vi "Teleop.vi"(10 "Match Info":T1={"Autonomous Elapsed Seconds"=0.0, "TeleOp Elapsed Seconds"=0.0, "Disabled Elapsed Seconds"=0.0, "Visited Autonomous"=FALSE, "Visited TeleOp"=FALSE, "Visited Disabled"=FALSE, "Autonomous Settings"={"Autonomous Style"=enum."Independent", "VI Refnum"=refnum}}, 11 "Call Context":T2) -> ()   [LabVIEW 2017]
doc: "This VI is called for each TeleOp packet received from the DS where the robot is not disabled. It is often used to read from the joysticks and update I/O or to update setpoints for timed control loops. It should complete and return within 20 milliseconds or it may miss DS packets."
uses:
  <vilib>/Rock Robotics/WPI/DriverStation/WPI_DriverStationDerivedRobotMode.ctl
  <vilib>/Rock Robotics/WPI/DriverStation/WPI_DriverStationMatch Info.ctl
  <vilib>/Rock Robotics/WPI/Solenoid/WPI_SolenoidValue.ctl
  <vilib>/Rock Robotics/WPI/ThirdParty/Phoenix-LabVIEW/Motor Controller/Controls/CTRE_Phoenix_MotorControl_ControlMode.ctl
  <vilib>/Rock Robotics/WPI/Utilities/WPI_GetSetVariantRefNum.vi
  <vilib>/Rock Robotics/WPI/Solenoid/WPI_SolenoidSetEnum.vi
  <vilib>/Rock Robotics/Network Tables/NT Write Boolean Array.vi
  <vilib>/Rock Robotics/Network Tables/NT Write Numeric Array.vi
  <vilib>/Rock Robotics/Network Tables/NT Read Boolean.vi
  <vilib>/Rock Robotics/Network Tables/NT Read Number.vi
  Robot Global Data.vi
  <vilib>/addons/control/pid/NI_PID_pid.lvlib
  <vilib>/addons/control/pid/pid.llb/PID (DBL).vi
panel:
  out "AbsArm":dbl
  out "Sample Slider 0":dbl(slide) scale=0.0..5.0
  out "Sample Boolean 1":bool
  out "Sample Boolean 0":bool
  # "TUSKS"
  # "Axis 1"
  # "DRIVE"
  # "Axis 1"
  # "PULSE"
  # "Button 3"
  # "Button 3"
  # "Axis 0"
  # "Axis 0"
  # "Button 2"
  # "Button 1"
  # "Button 2"
  # "Button 1"
  # "Button 0"
  # "Button 0"
  # "CONTROLLER  LAYOUT"
  # "CONTROLLER  LAYOUT"
  # "Joystick 1"
  # "Joystick 0"
  # "Joystick 1"
  # "https://www.xbox.com/en-us/xbox-one/accessories"
  # "Axis 4"
  # "Axis 4"
  # "DRIVE TURN"
  # "Left"
  # "Left"
  # "Axis 5"
  # "Axis 5"
  # "CLAW IN"
  # "Button 4"
  # "ELBOW DOWN"
  # "Button 4"
  # "Axis 2"
  # "ARM DOWN"
  # "Axis 2"
  # "BELT IN"
  # "Right"
  # "Button 5"
  # "ELBOW UP"
  # "Button 5"
  # "CLAW OUT"
  # "Axis 3"
  # "ARM UP"
  # "Axis 3"
  # "BELT OUT"
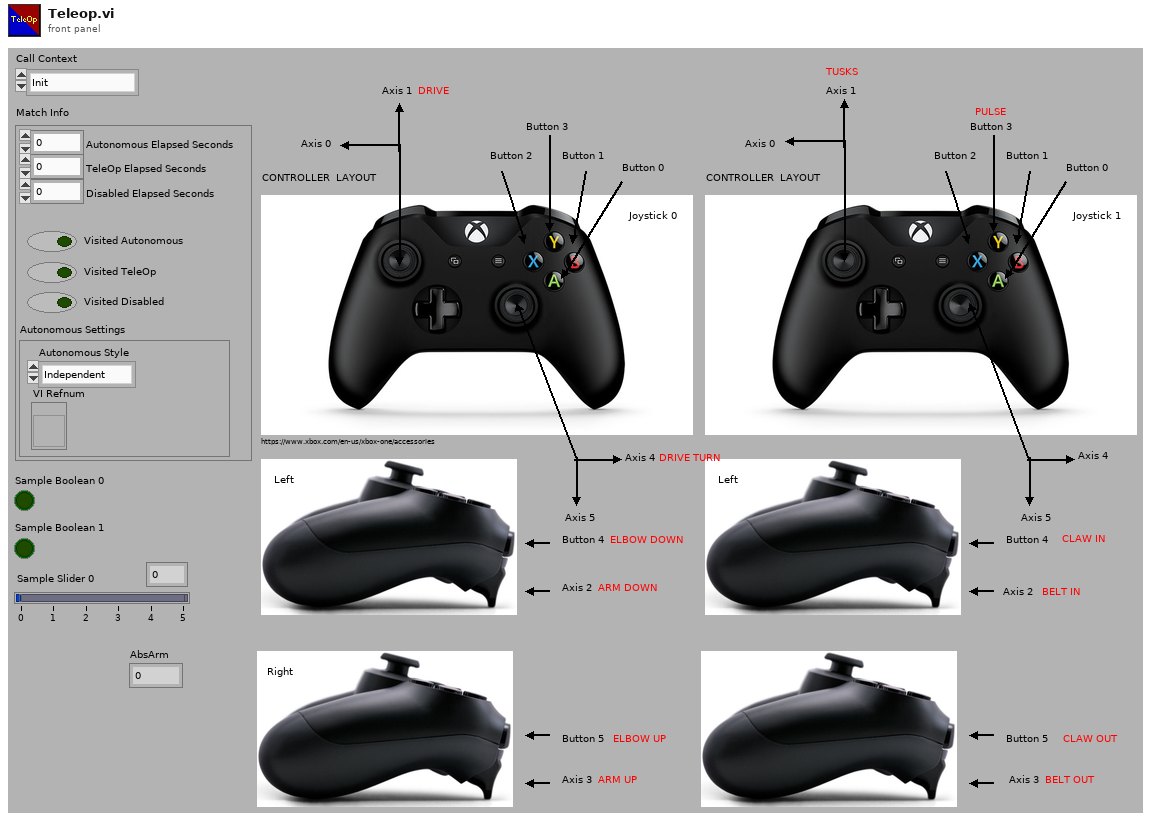
[diagram p1: front panel]
types:
  T1 = typedef "WPI_DriverStationMatch Info.ctl" = cluster{"Autonomous Elapsed Seconds":dbl, "TeleOp Elapsed Seconds":dbl, "Disabled Elapsed Seconds":dbl, "Visited Autonomous":bool, "Visited TeleOp":bool, "Visited Disabled":bool, "Autonomous Settings":cluster{"Autonomous Style":enum16{"Iterative", "Independent"}, "VI Refnum":refnum<vi>}}
  T2 = typedef "WPI_DriverStationDerivedRobotMode.ctl" = enum16{"Init", "Execute", "Stop"}
  T3 = typedef "WPI_JoystickDevRef.ctl" = cluster{"Device":T4}
  T4 = typedef "WPI_JoystickDeviceEnum.ctl" = enum16{"USB 0", "USB 1", "USB 2", "USB 3", "USB 4", "USB 5"}
  T5 = cluster{"Axes[0]":dbl, "Axes[1]":dbl, "Axes[2]":dbl, "Axes[3]":dbl, "Axes[4]":dbl, "Axes[5]":dbl, "Axes[6]":dbl, "Axes[7]":dbl, "Axes[8]":dbl}
  T6 = cluster{"Buttons[0]":bool, "Buttons[1]":bool, "Buttons[2]":bool, "Buttons[3]":bool, "Buttons[4]":bool, "Buttons[5]":bool, "Buttons[6]":bool, "Buttons[7]":bool, "Buttons[8]":bool}
  T7 = typedef "CTRE_Phoenix_MotorControl_ControlMode.ctl" = u16
  T8 = typedef "WPI_MotorControlDeviceRef.ctl" = cluster{"DeviceStatus":errorcluster, "Type":T9, "PWM":cluster{"PWM Channel":T10, "DeadBand":T11}, "CAN":cluster{"Device Number":u8, "SetOutput VI Ref":variant, "GetOutput VI Ref":variant, "Enable VI Ref":variant, "Disable VI Ref":variant, "Data":variant}, "Invert":bool, "DIO PWM":cluster{"PWM \"Enable\" Channel":T10, "DIOChannel":T12, "PWM Rate":dbl}}
  T9 = typedef "WPI_MotorControlType.ctl" = enum16{"PWM", "CAN", "DIO PWM"}
  T10 = typedef "FPGA_DIOPWMChannel.ctl" = enum8{"PWM 0", "PWM 1", "PWM 2", "PWM 3", "PWM 4", "PWM 5", "PWM 6", "PWM 7", "PWM 8", "PWM 9", "PWM MXP 0", "PWM MXP 1", "PWM MXP 2", "PWM MXP 3", "PWM MXP 4", "PWM MXP 5", "PWM MXP 6", "PWM MXP 7", "PWM MXP 8", "PWM MXP 9", "Invalid"}
  T11 = typedef "WPI_PWMDeadband.ctl" = cluster{"Name":string, "maxPositivePwm":i32, "minPositivePwm":i32, "centerPwm":i32, "maxNegativePwm":i32, "minNegativePwm":i32, "angularRange":u16}
  T12 = typedef "FPGA_DIOChannel.ctl" = enum8{"DIO 0", "DIO 1", "DIO 2", "DIO 3", "DIO 4", "DIO 5", "DIO 6", "DIO 7", "DIO 8", "DIO 9", "DIO MXP 0", "DIO MXP 1", "DIO MXP 2", "DIO MXP 3", "DIO MXP 4", "DIO MXP 5", "DIO MXP 6", "DIO MXP 7", "DIO MXP 8", "DIO MXP 9", "DIO MXP 10", "DIO MXP 11", "DIO MXP 12", "DIO MXP 13", "DIO MXP 14", "DIO MXP 15", "SPI Port CS1", "SPI Port CS2", "SPI Port CS3", "SPI Port MISO", "SPI Port MOSI", "Invalid"}
  T13 = enum16{"Arm Down", "Arm Switch", "Arm(Low Scale)", "Arm(Normal Scale)", "Arm(High Scale)", "Hang"}
  T14 = cluster{"proportional gain (Kc)":dbl, "integral time (Ti, min)":dbl, "derivative time (Td, min)":dbl}
  T15 = enum16{"Arm Down", "Arm Switch", "Arm(Low Scale)", "Arm(Normal Scale)", "Arm(High Scale)"}
  T16 = typedef "WPI_SolenoidValue.ctl" = enum16{"Off", "On", "Forward", "Reverse"}
  T17 = typedef "WPI_SolenoidDevRef.ctl" = cluster{"DevStatus":errorcluster, "Pneumatics Control Module":u8, "Forward Solenoid Channel":T18, "Reverse Solenoid Channel":T18}
  T18 = typedef "WPI_SolenoidChannel.ctl" = enum8{"Solenoid 0", "Solenoid 1", "Solenoid 2", "Solenoid 3", "Solenoid 4", "Solenoid 5", "Solenoid 6", "Solenoid 7", "Invalid"}
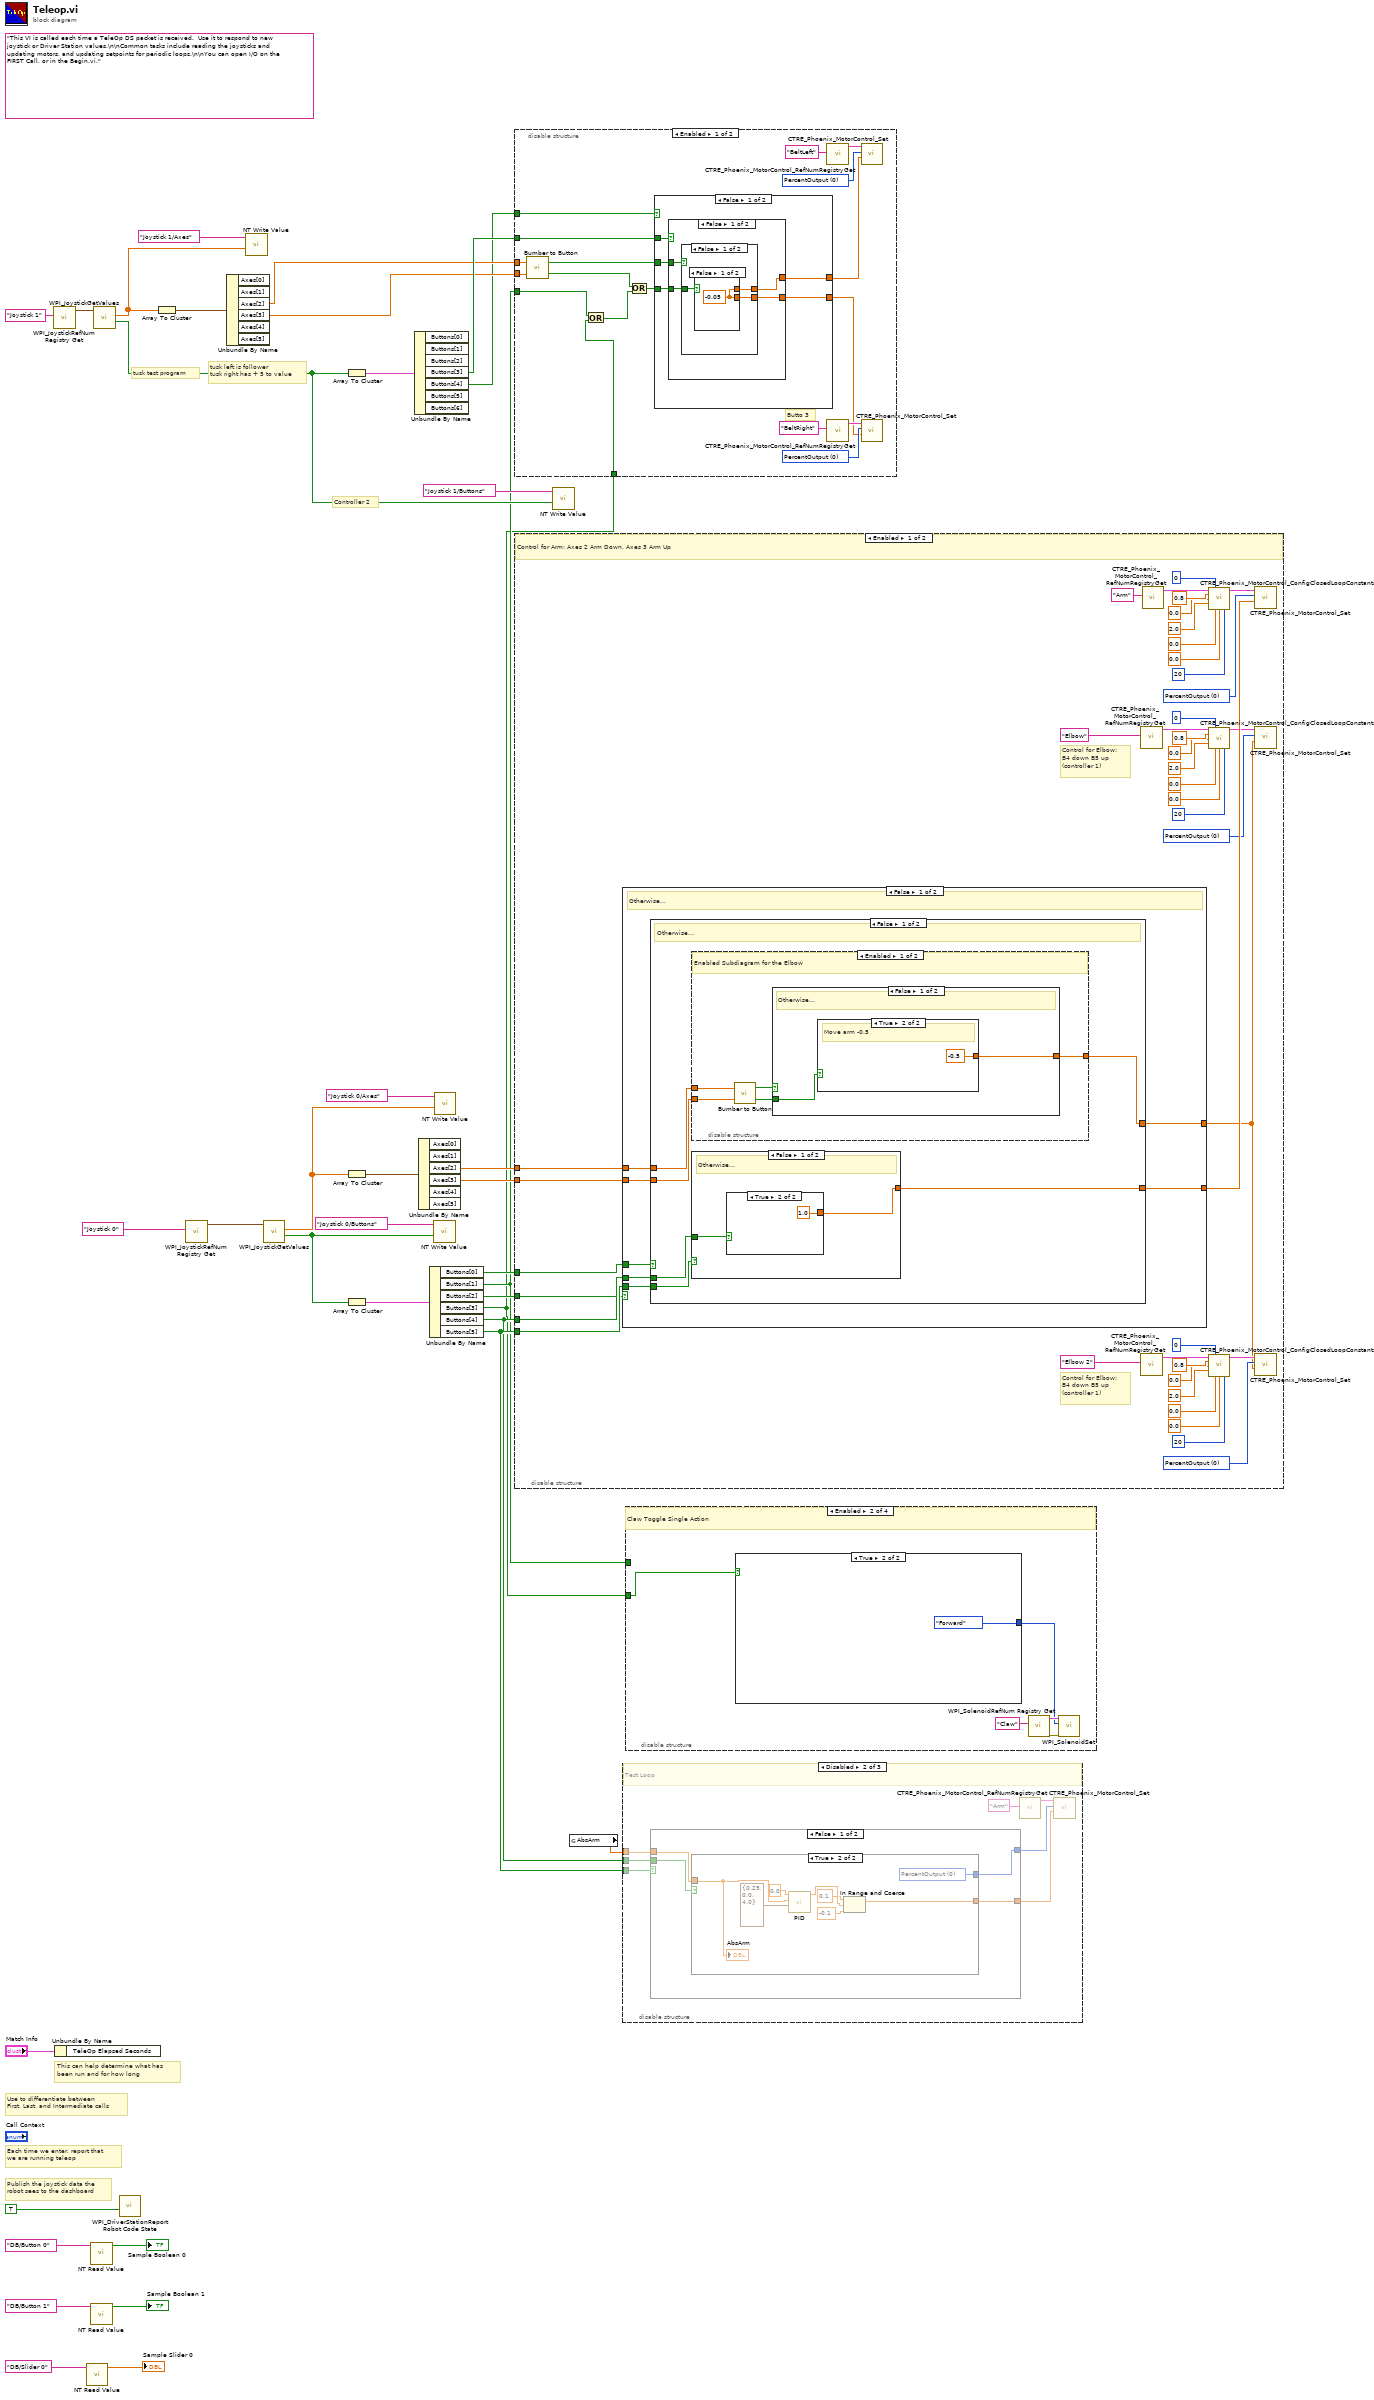
[diagram p0: block diagram]
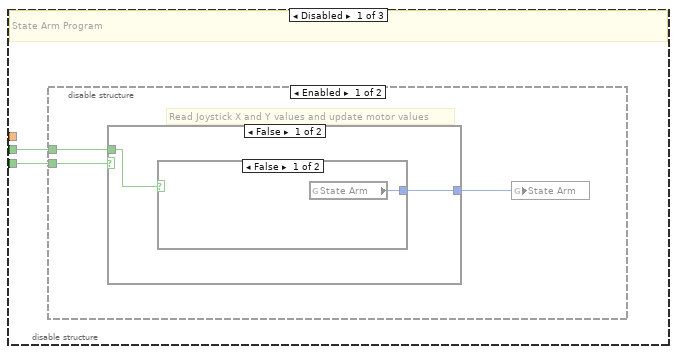
[diagram p2: hidden frame]
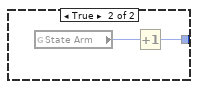
[diagram p3: hidden frame]
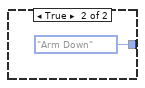
[diagram p4: hidden frame]
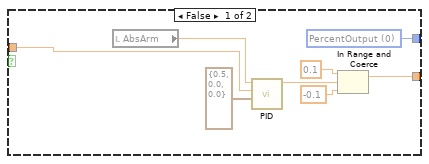
[diagram p6: hidden frame]
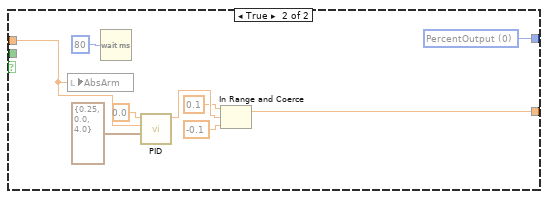
[diagram p7: hidden frame]
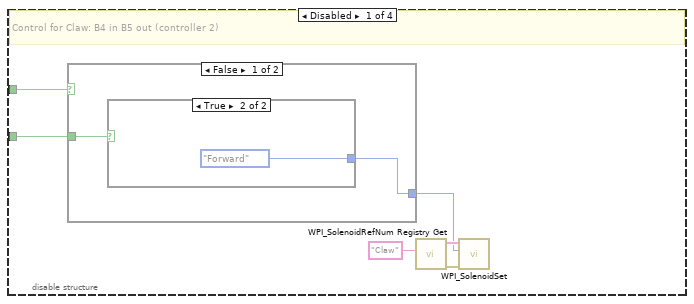
[diagram p9: hidden frame]
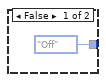
[diagram p10: hidden frame]
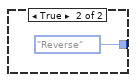
[diagram p11: hidden frame]
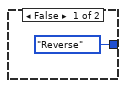
[diagram p12: hidden frame]
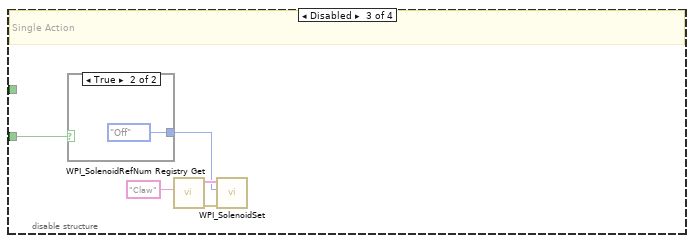
[diagram p13: hidden frame]
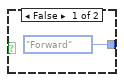
[diagram p14: hidden frame]
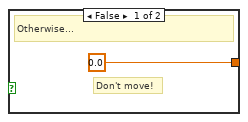
[diagram p16: hidden frame]
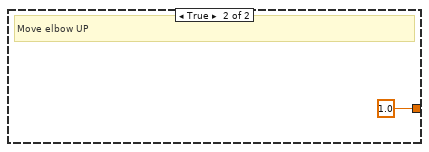
[diagram p17: hidden frame]
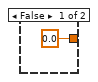
[diagram p19: hidden frame]
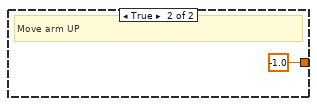
[diagram p20: hidden frame]
diagram:
  (unwired) "This VI is called each time a TeleOp DS packet is received.  Use it to respond to new joystick or Driver Station values.\n\nCommon tasks include reading the joysticks and updating motors, and updating setpoints for periodic loops.\n\nYou can open I/O on the FIRST Call, or in the Begin.vi."
  # "tusk left is follower\ntusk right has + 5 to value"
  # "tusk test program"
  # "Controller 2"
  # "Publish the joystick data the\nrobot sees to the dashboard"
  # "Each time we enter, report that\nwe are running teleop"
  # "Use to differentiate between\nFirst, Last, and Intermediate calls"
  # "This can help determine what has\nbeen run and for how long"
  n1 = call <vilib>:"WPI_JoystickRefNum Registry Get.vi"("refnum name"="Joystick 1") -> ("JoystickDevRef"=w21:T3)  [unwired: 9 in, 1 out]
  n2 = Unbundle By Name("Match Info") -> ()  [unwired: 1 out]
  n3 = call-poly <vilib>:"NT Read Value.vi"("Name"="DB/Slider 0" ("refnum name")) -> ("Numeric"=→"Sample Slider 0":dbl)  [unwired: 9 in, 1 out]
  n4 = call-poly <vilib>:"NT Read Value.vi"("Name"="DB/Button 0" ("refnum name")) -> ("Boolean"=→"Sample Boolean 0":bool)  [unwired: 9 in, 1 out]
  n5 = call-poly <vilib>:"NT Read Value.vi"("Name"="DB/Button 1" ("refnum name")) -> ("Boolean"=→"Sample Boolean 1":bool)  [unwired: 9 in, 1 out]
  n6 = call <vilib>:"WPI_JoystickGetValues.vi"("JoystickDevRef"=w21) -> ("Buttons"=w16:bool[], "Axes"=w15:dbl[])  [unwired: 6 in, 3 out]
  n7 = call <vilib>:"WPI_DriverStationReport Robot Code State.vi"("TeleOp"=TRUE ("Autonomous")) -> ()  [unwired: 10 in, 1 out]
  n8 = Array To Cluster(array=w15) -> (cluster=w19:T5)
  n9 = call <vilib>:"WPI_JoystickRefNum Registry Get.vi"("refnum name"="Joystick 0") -> ("JoystickDevRef"=w35:T3)  [unwired: 1 in, 9 out]
  n10 = Unbundle By Name(w19) -> ("Axes[2]"=w11:dbl, "Axes[3]"=w12:dbl)  [unwired: 4 out]
  n11 = call-poly <vilib>:"NT Write Value.vi"("Numeric Array"=w15, "Name"="Joystick 1/Axes") -> ()  [unwired: 9 in, 1 out]
  n12 = call <vilib>:"WPI_JoystickGetValues.vi"("JoystickDevRef"=w35) -> ("Buttons"=w23:bool[], "Axes"=w25:dbl[])  [unwired: 6 in, 3 out]
  n13 = Array To Cluster(array=w16) -> (cluster=w18:T6)
  n14 = Array To Cluster(array=w25) -> (cluster=w24:T5)
  n15 = Array To Cluster(array=w23) -> (cluster=w22:T6)
  n16 = Unbundle By Name(w18) -> ("Buttons[3]"=w13:bool, "Buttons[4]"=w3:bool)  [unwired: 5 out]
  n17 = Unbundle By Name(w24) -> ("Axes[2]"=w6:dbl, "Axes[3]"=w5:dbl)  [unwired: 4 out]
  n18 = Unbundle By Name(w22) -> ("Buttons[0]"=w4:bool, "Buttons[1]"=w2:bool, "Buttons[2]"=w9:bool, "Buttons[3]"=w1:bool, "Buttons[4]"=w7:bool, "Buttons[5]"=w8:bool)
  n19 = call-poly <vilib>:"NT Write Value.vi"("Boolean Array"=w23, "Name"="Joystick 0/Buttons") -> ()  [unwired: 9 in, 1 out]
  n20 = call-poly <vilib>:"NT Write Value.vi"("Numeric Array"=w25, "Name"="Joystick 0/Axes") -> ()  [unwired: 9 in, 1 out]
  n21 = disable-structure shown="Enabled" {
    disable-tunnel: w13 -> [w48 _]
    disable-tunnel: w12 -> [w47 _]
    disable-tunnel: w11 -> [w46 _]
    disable-tunnel: w3 -> [w45 _]
    disable-tunnel: w2 -> [w39 _]
    disable-tunnel: w1 -> [w40 _]
    frame Enabled {
      w50 = T7 0 items=["PercentOutput"=0, "Position"=1, "Velocity"=2, "Current"=3, "Follower"=5, "MotionProfile"=6, "MotionMagic"=7, "MotionMagicArc"=8, "MotionProfileArc"=10, "Disabled"=15] ("Control Mode")
      w51 = T7 0 items=["PercentOutput"=0, "Position"=1, "Velocity"=2, "Current"=3, "Follower"=5, "MotionProfile"=6, "MotionMagic"=7, "MotionMagicArc"=8, "MotionProfileArc"=10, "Disabled"=15] ("Control Mode")
      # "Butto 3"
      n22 = call "Bumber to Button.vi"("Bumper / Axis 2"=w47, "Bumper / Axis 1"=w46) -> ("Boolean Output 2"=w42:bool, "Boolean Output 1"=w41:bool)
      n23 = Or(x=w39, y=w40) -> (x .or. y?=w38:bool)
      n24 = Or(x=w42, y=w38) -> (x .or. y?=w43:bool)
      n25 = case shown="False" w45 {
        tunnel: [w60 w73] -> w44
        tunnel: [w59 w73] -> w49
        tunnel: w48 -> [w58 _]
        tunnel: w41 -> [w57 _]
        tunnel: w43 -> [w56 _]
        frame False {
          n26 = case shown="False" w58 {
            tunnel: [w64 1.0 ("Output")] -> w59
            tunnel: [w63 -1.0 ("Output")] -> w60
            tunnel: w57 -> [w62 _]
            tunnel: w56 -> [w61 _]
            frame False {
              n27 = case shown="False" w62 {
                tunnel: [w67 w70] -> w64
                tunnel: [w66 w70] -> w63
                tunnel: w61 -> [w65 _]
                frame False {
                  n28 = case shown="False" w65 {
                    tunnel: [w68 w69] -> w67
                    tunnel: [w68 w69] -> w66
                    frame False {
                      w68 = -0.05 ("Output")
                    }
                    frame True {
                      w69 = -1.0 ("Output")
                    }
                  }
                }
                frame True {
                  w70 = 1.0 ("Output")
                }
              }
            }
            frame True {
              # "Pulse"
            }
          }
        }
        frame True {
          w73 = 0.3 ("Output")
        }
      }
      n29 = call <vilib>:"CTRE_Phoenix_MotorControl_RefNumRegistryGet.vi"("refnum name"="BeltLeft") -> ("PhoenixMotorControlDevRef"=w55:T8)  [unwired: 9 in, 1 out]
      n30 = call <vilib>:"CTRE_Phoenix_MotorControl_RefNumRegistryGet.vi"("refnum name"="BeltRight") -> ("PhoenixMotorControlDevRef"=w54:T8)  [unwired: 9 in, 1 out]
      n31 = call <vilib>:"CTRE_Phoenix_MotorControl_Set.vi"("Output"=w49, "Control Mode"=w50, "PhoenixMotorControlDevRef"=w55) -> ()  [unwired: 7 in, 2 out]
      n32 = call <vilib>:"CTRE_Phoenix_MotorControl_Set.vi"("Output"=w44, "Control Mode"=w51, "PhoenixMotorControlDevRef"=w54) -> ()  [unwired: 7 in, 2 out]
    }
    frame Disabled {
    }
  }
  n33 = disable-structure "Diagram Disable Structure" shown="Enabled" {
    disable-tunnel: w9 -> [w86 _]
    disable-tunnel: w8 -> [w103 _]
    disable-tunnel: w7 -> [w102 _]
    disable-tunnel: w6 -> [w99 _]
    disable-tunnel: w5 -> [w100 _]
    disable-tunnel: w4 -> [w87 _]
    frame Enabled {
      w76 = T7 0 items=["PercentOutput"=0, "Position"=1, "Velocity"=2, "Current"=3, "Follower"=5, "MotionProfile"=6, "MotionMagic"=7, "MotionMagicArc"=8, "MotionProfileArc"=10, "Disabled"=15] ("Control Mode")
      w89 = T7 0 items=["PercentOutput"=0, "Position"=1, "Velocity"=2, "Current"=3, "Follower"=5, "MotionProfile"=6, "MotionMagic"=7, "MotionMagicArc"=8, "MotionProfileArc"=10, "Disabled"=15] ("Control Mode")
      w113 = T7 0 items=["PercentOutput"=0, "Position"=1, "Velocity"=2, "Current"=3, "Follower"=5, "MotionProfile"=6, "MotionMagic"=7, "MotionMagicArc"=8, "MotionProfileArc"=10, "Disabled"=15] ("Control Mode")
      # "Control for Elbow:\nB4 down B5 up\n(controller 1)"
      # "Control for Elbow:\nB4 down B5 up\n(controller 1)"
      # "Control for Arm: Axes 2 Arm Down, Axes 3 Arm Up"
      n34 = case shown="False" w86 {
        tunnel: w87 -> [w121 _]
        tunnel: w103 -> [w120 _]
        tunnel: w102 -> [w119 _]
        tunnel: [w118 0.7 ("Output")] -> w101
        tunnel: w100 -> [w117 _]
        tunnel: w99 -> [w116 _]
        tunnel: [w115 -1.0 ("Output")] -> w74
        frame False {
          # "Otherwise..."
          n35 = case shown="False" w121 {
            tunnel: w120 -> [w127 _]
            tunnel: w119 -> [w126 _]
            tunnel: [w125 -0.7 ("Output")] -> w118
            tunnel: w117 -> [w123 _]
            tunnel: w116 -> [w124 _]
            tunnel: [w122 1.0 ("Output")] -> w115
            frame False {
              # "Otherwise..."
              n36 = disable-structure "Diagram Disable Structure" shown="Enabled" {
                disable-tunnel: w124 -> [w130 _]
                disable-tunnel: w123 -> [w129 _]
                disable-tunnel: [w128 _] -> w122
                frame Enabled {
                  # "Enabled Subdiagram for the Elbow"
                  n37 = call "Bumber to Button.vi"("Bumper / Axis 2"=w129, "Bumper / Axis 1"=w130) -> ("Boolean Output 2"=w131:bool, "Boolean Output 1"=w132:bool)
                  n38 = case shown="False" w132 {
                    tunnel: [w134 1.0 ("Output")] -> w128
                    tunnel: w131 -> [w133 _]
                    frame False {
                      # "Otherwise..."
                      n39 = case shown="True" w133 {
                        tunnel: [0.0 ("Output") -0.5 ("Output")] -> w134
                        frame False {
                          # "Don't move!"
                          # "Otherwise..."
                        }
                        frame True {
                          # "Move arm -0.5"
                        }
                      }
                    }
                    frame True {
                      # "Move elbow UP"
                    }
                  }
                }
                frame Disabled {
                  # "Disabled Elbow diagram"
                }
              }
              n40 = case shown="False" w127 {
                tunnel: [w139 -1.0 ("Output")] -> w125
                tunnel: w126 -> [w138 _]
                frame False {
                  # "Otherwise..."
                  n41 = case shown="True" w138 {
                    tunnel: [0.0 ("Output") 1.0 ("Output")] -> w139
                    frame False {
                    }
                    frame True {
                    }
                  }
                }
                frame True {
                  # "Move arm UP"
                }
              }
            }
            frame True {
              # "Move arm 1 and elbow -0.6  (same speed)"
            }
          }
        }
        frame True {
          # "If true, arm -1, elbow 0.6 (same speed)"
        }
      }
      n42 = call <vilib>:"CTRE_Phoenix_MotorControl_RefNumRegistryGet.vi"("refnum name"="Elbow") -> ("PhoenixMotorControlDevRef"=w97:T8)  [unwired: 9 in, 1 out]
      n43 = call <vilib>:"CTRE_Phoenix_MotorControl_RefNumRegistryGet.vi"("refnum name"="Elbow 2") -> ("PhoenixMotorControlDevRef"=w84:T8)  [unwired: 9 in, 1 out]
      n44 = call <vilib>:"CTRE_Phoenix_MotorControl_RefNumRegistryGet.vi"("refnum name"="Arm") -> ("PhoenixMotorControlDevRef"=w112:T8)  [unwired: 9 in, 1 out]
      n45 = call <vilib>:"CTRE_Phoenix_MotorControl_ConfigClosedLoopConstants.vi"("PhoenixMotorControlDevRef"=w112, "slotIdx"=0, "P"=0.8, "I"=0.0, "D"=2.0, "F"=0.0, "I Zone"=0.0, "timeoutMs"=20) -> ("PhoenixMotorControlDevRef"=w111:T8)  [unwired: 6 in, 1 out]
      n46 = call <vilib>:"CTRE_Phoenix_MotorControl_ConfigClosedLoopConstants.vi"("PhoenixMotorControlDevRef"=w97, "slotIdx"=0, "P"=0.8, "I"=0.0, "D"=2.0, "F"=0.0, "I Zone"=0.0, "timeoutMs"=20) -> ("PhoenixMotorControlDevRef"=w98:T8)  [unwired: 6 in, 1 out]
      n47 = call <vilib>:"CTRE_Phoenix_MotorControl_ConfigClosedLoopConstants.vi"("PhoenixMotorControlDevRef"=w84, "slotIdx"=0, "P"=0.8, "I"=0.0, "D"=2.0, "F"=0.0, "I Zone"=0.0, "timeoutMs"=20) -> ("PhoenixMotorControlDevRef"=w85:T8)  [unwired: 6 in, 1 out]
      n48 = call <vilib>:"CTRE_Phoenix_MotorControl_Set.vi"("Output"=w101, "Control Mode"=w113, "PhoenixMotorControlDevRef"=w111) -> ()  [unwired: 7 in, 2 out]
      n49 = call <vilib>:"CTRE_Phoenix_MotorControl_Set.vi"("Output"=w74, "Control Mode"=w89, "PhoenixMotorControlDevRef"=w98) -> ()  [unwired: 7 in, 2 out]
      n50 = call <vilib>:"CTRE_Phoenix_MotorControl_Set.vi"("Output"=w74, "Control Mode"=w76, "PhoenixMotorControlDevRef"=w85) -> ()  [unwired: 7 in, 2 out]
    }
    frame Disabled {
      # "Arm Disabled"
    }
  }
  n51 = call-poly <vilib>:"NT Write Value.vi"("Boolean Array"=w16, "Name"="Joystick 1/Buttons") -> ()  [unwired: 9 in, 1 out]
  n52 = global read "Robot Global Data.vi" "AbsArm"() -> (w10:dbl)
  n53 = disable-structure shown="Disabled" {
    disable-tunnel: w10 -> [_ w162 _]
    disable-tunnel: w7 -> [w147 w159 _]
    disable-tunnel: w8 -> [w148 w158 _]
    frame Disabled {
      # "State Arm Program"
      n54 = disable-structure shown="Enabled" {
        disable-tunnel: w148 -> [w150 _]
        disable-tunnel: w147 -> [w149 _]
        frame Enabled {
          # "Read Joystick X and Y values and update motor values"
          n55 = case shown="False" w150 {
            tunnel: [w153 T13."Arm Down" ("State Arm")] -> w151
            tunnel: w149 -> [w152 _]
            frame False {
              n56 = case shown="False" w152 {
                tunnel: [w154 w155] -> w153
                frame False {
                  n57 = global read "Robot Global Data.vi" "State Arm"() -> (w154:T15)
                }
                frame True {
                  n58 = global read "Robot Global Data.vi" "State Arm"() -> (w156:T15)
                  n59 = Increment(x=w156) -> (x+1=w155:T15)
                }
              }
            }
            frame True {
            }
          }
          n60 = global write "Robot Global Data.vi" "State Arm"(w151) -> ()
        }
        frame Disabled {
        }
      }
    }
    frame Disabled {
      # "Test Loop"
      n61 = case shown="False" w158 {
        tunnel: [w168 w187] -> w160
        tunnel: [w166 w186] -> w161
        tunnel: w162 -> [w167 w185]
        tunnel: w159 -> [w165 _]
        frame False {
          n62 = case shown="True" w165 {
            tunnel: [w176 w180] -> w166
            tunnel: [w173 w179] -> w168
            tunnel: w167 -> [w170 w177]
            frame False {
              w176 = T7 0 items=["PercentOutput"=0, "Position"=1, "Velocity"=2, "Current"=3, "Follower"=5, "MotionProfile"=6, "MotionMagic"=7, "MotionMagicArc"=8, "MotionProfileArc"=10, "Disabled"=15] ("Control Mode")
              n63 = local read "AbsArm"() -> (w169:dbl)
              n64 = call-poly <vilib>:"PID.vi"("PID gains"=T14 {"proportional gain (Kc)"=0.5, "integral time (Ti, min)"=0.0, "derivative time (Td, min)"=0.0}, "process variable"=w170, "setpoint"=w169) -> ("output"=w171:dbl)  [unwired: 7 in, 1 out]
              n65 = In Range and Coerce(upper limit=0.1, x=w171, lower limit=-0.1) -> (coerced(x)=w173:dbl)  [unwired: 1 out]
            }
            frame True {
              w180 = T7 0 items=["PercentOutput"=0, "Position"=1, "Velocity"=2, "Current"=3, "Follower"=5, "MotionProfile"=6, "MotionMagic"=7, "MotionMagicArc"=8, "MotionProfileArc"=10, "Disabled"=15] ("Control Mode")
              n66 = call-poly <vilib>:"PID.vi"("PID gains"=T14 {"proportional gain (Kc)"=0.25, "integral time (Ti, min)"=0.0, "derivative time (Td, min)"=4.0}, "process variable"=w177, "setpoint"=0.0) -> ("output"=w184:dbl)  [unwired: 7 in, 1 out]
              n67 = In Range and Coerce(upper limit=0.1, x=w184, lower limit=-0.1) -> (coerced(x)=w179:dbl)  [unwired: 1 out]
              "AbsArm" <- w177
            }
          }
        }
        frame True {
          w186 = T7 0 items=["PercentOutput"=0, "Position"=1, "Velocity"=2, "Current"=3, "Follower"=5, "MotionProfile"=6, "MotionMagic"=7, "MotionMagicArc"=8, "MotionProfileArc"=10, "Disabled"=15] ("Control Mode")
          n68 = local write "AbsArm"(w185) -> ()
          n69 = Wait (ms)(milliseconds to wait=u32 80) -> ()  [unwired: 1 out]
          n70 = call-poly <vilib>:"PID.vi"("PID gains"=T14 {"proportional gain (Kc)"=0.25, "integral time (Ti, min)"=0.0, "derivative time (Td, min)"=4.0}, "process variable"=w185, "setpoint"=0.0) -> ("output"=w190:dbl)  [unwired: 7 in, 1 out]
          n71 = In Range and Coerce(upper limit=0.1, x=w190, lower limit=-0.1) -> (coerced(x)=w187:dbl)  [unwired: 1 out]
        }
      }
      n72 = call <vilib>:"CTRE_Phoenix_MotorControl_RefNumRegistryGet.vi"("refnum name"="Arm") -> ("PhoenixMotorControlDevRef"=w163:T8)  [unwired: 9 in, 1 out]
      n73 = call <vilib>:"CTRE_Phoenix_MotorControl_Set.vi"("Output"=w160, "Control Mode"=w161, "PhoenixMotorControlDevRef"=w163) -> ()  [unwired: 7 in, 2 out]
    }
    frame Enabled {
      # "Arm Presets Disabled"
    }
  }
  n74 = disable-structure "Diagram Disable Structure" shown="Enabled" {
    disable-tunnel: w1 -> [w196 w206 w212 _]
    disable-tunnel: w2 -> [w194 _ _ _]
    frame Disabled {
      # "Control for Claw: B4 in B5 out (controller 2)"
      n75 = case shown="False" w194 {
        tunnel: w196 -> [w201 _]
        tunnel: [w200 WPI_SolenoidValue."Reverse" ("Value")] -> w195
        frame False {
          n76 = case shown="True" w201 {
            tunnel: [WPI_SolenoidValue."Off" ("Value") WPI_SolenoidValue."Forward" ("Value")] -> w200
            frame False {
            }
            frame True {
            }
          }
        }
        frame True {
        }
      }
      n77 = call <vilib>:"WPI_SolenoidRefNum Registry Get.vi"("refnum name"="Claw") -> ("error out"=w198:errorcluster, "SolenoidDevRef"=w199:T17)  [unwired: 9 in]
      n78 = call-poly <vilib>:"WPI_SolenoidSet.vi"("error in (no error)"=w198, "Value"=w195, "SolenoidDevRef"=w199) -> ()  [unwired: 7 in, 2 out]
    }
    frame Enabled {
      # "Claw Toggle Single Action"
      n79 = case shown="True" w206 {
        tunnel: [WPI_SolenoidValue."Reverse" ("Value") WPI_SolenoidValue."Forward" ("Value")] -> w205
        frame False {
        }
        frame True {
        }
      }
      n80 = call <vilib>:"WPI_SolenoidRefNum Registry Get.vi"("refnum name"="Claw") -> ("error out"=w208:errorcluster, "SolenoidDevRef"=w209:T17)  [unwired: 9 in]
      n81 = call-poly <vilib>:"WPI_SolenoidSet.vi"("error in (no error)"=w208, "Value"=w205, "SolenoidDevRef"=w209) -> ()  [unwired: 7 in, 2 out]
    }
    frame Disabled {
      # "Single Action"
      n82 = case shown="True" w212 {
        tunnel: [WPI_SolenoidValue."Forward" ("Value") WPI_SolenoidValue."Off" ("Value")] -> w213
        frame False {
        }
        frame True {
        }
      }
      n83 = call <vilib>:"WPI_SolenoidRefNum Registry Get.vi"("refnum name"="Claw") -> ("error out"=w215:errorcluster, "SolenoidDevRef"=w216:T17)  [unwired: 9 in]
      n84 = call-poly <vilib>:"WPI_SolenoidSet.vi"("error in (no error)"=w215, "Value"=w213, "SolenoidDevRef"=w216) -> ()  [unwired: 7 in, 2 out]
    }
    frame Disabled {
      # "Claw Disabled"
    }
  }
